vi "GetAllTemplates.vi"(4 "Category Nonlocalized Names":string[](array[string]), 6 "Category Names":string[](array[string])) -> (3 "Templates Out":refnum<class "MetaDataObj.lvclass">[](array[class]))   [LabVIEW 2016, in "NI_NPW_Loading Project Info.lvlib"]
uses:
  <resource>/dialog/NewProjectWizard/Loading Project Info/NI_NPW_Loading Project Info.lvlib
  <resource>/dialog/NewProjectWizard/MetaDataObj/MetaDataObj.lvclass
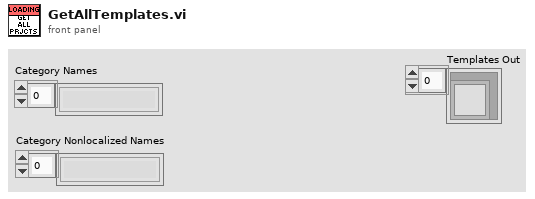
[diagram p1: front panel]
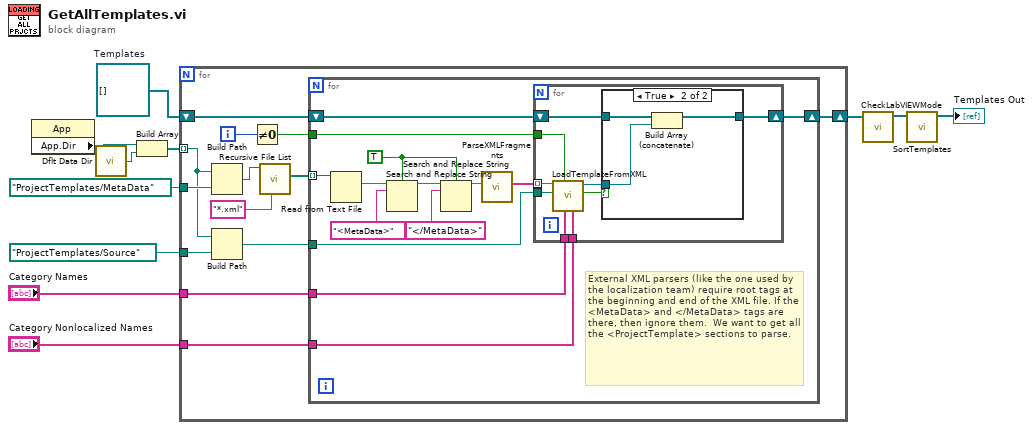
[diagram p0: block diagram]
diagram:
  w11 = refnum<class "MetaDataObj.lvclass">[] []  # Templates
  n1 = property class="App"() -> ("App.Dir"=w3:path)  [unwired: 2 in, 2 out]
  n2 = call <vilib>:"Dflt Data Dir.vi"() -> ("App:Default Data Directory"=w7:path)
  n3 = Build Array(w3, w7) -> (w6:path[])
  n4 = for {
    tunnel: w6 -> [w21] mode=indexing
    shift-right: [w23] -> w9
    shift-left: w11 -> [w24]
    tunnel: path "ProjectTemplates/MetaData" -> [w22]
    tunnel: path "ProjectTemplates/Source" -> [w20]
    tunnel: "Category Names" -> [w13]
    tunnel: "Category Nonlocalized Names" -> [w12]
    i -> [w15]
    n5 = Build Path(base path=w21, name or relative path=w22) -> (appended path=w19:path)
    n6 = Build Path(base path=w21, name or relative path=w20) -> (appended path=w16:path)
    n7 = Not Equal To 0?(x=w15) -> (x != 0?=w14:bool)
    n8 = call <vilib>:"Recursive File List.vi"("pattern"="*.xml", "Folder Path"=w19) -> ("All Files in Dir"=w17:path[])  [unwired: 5 in, 4 out]
    n9 = for {
      shift-right: [w28] -> w23
      shift-left: w24 -> [w29]
      tunnel: w17 -> [w38] mode=indexing
      tunnel: w16 -> [w37]
      tunnel: w14 -> [w27]
      tunnel: w13 -> [w26]
      tunnel: w12 -> [w25]
      w33 = TRUE ("ignore case? (F)")
      # "External XML parsers (like the one used by the localization team) require root tags at the beginning and end of the XML file. If the <MetaData> and </MetaData> tags are there, then ignore them.  We want to get all the <ProjectTemplate> sections to parse."
      n10 = Read from Text File(file (use dialog)=w38) -> (text=w35:string)  [unwired: 3 in, 3 out]
      n11 = Search and Replace String(case sensitive?=w33, input string=w35, search string="<MetaData>") -> (result string=w34:string)  [unwired: 5 in, 3 out]
      n12 = Search and Replace String(case sensitive?=w33, input string=w34, search string="</MetaData>") -> (result string=w31:string)  [unwired: 5 in, 3 out]
      n13 = call <vilib>:"ParseXMLFragments.vi"("XML in"=w31) -> ("XML Elements"=w36:string[])  [unwired: 9 in, 1 out]
      n14 = for {
        tunnel: w36 -> [w47] mode=indexing
        tunnel: w37 -> [w46]
        shift-right: [w43] -> w28
        shift-left: w29 -> [w44]
        tunnel: w27 -> [w41]
        tunnel: w26 -> [w40]
        tunnel: w25 -> [w39]
        n15 = call <resource>:"LoadTemplateFromXML.vi"("Category Nonlocalized Names"=w39, "Category Names"=w40, "Project Version Check? (F)"=w41, "Template Source Path"=w46, "XML String In"=w47) -> ("Valid Template?"=w42:bool, "Template Out"=w45:refnum<class "MetaDataObj.lvclass">)  [unwired: 5 in]
        n16 = case shown="True" w42 {
          tunnel: w45 -> [_ w49]
          tunnel: w44 -> [w48 w51]
          tunnel: [w48 w50] -> w43
          frame False {
          }
          frame True {
            n17 = Build Array (concatenate)(w51, w49) -> (w50:refnum<class "MetaDataObj.lvclass">[])
          }
        }
      }
    }
  }
  n18 = call <resource>:"CheckLabVIEWMode.vi"("Templates In"=w9) -> ("Templates Out"=w8:refnum<class "MetaDataObj.lvclass">[])  [unwired: 10 in]
  n19 = call <resource>:"SortTemplates.vi"("Unsorted Templates"=w8) -> ("Sorted Templates"=→"Templates Out":refnum<class "MetaDataObj.lvclass">[])  [unwired: 10 in]
